vi "Check mtcdt check cell radio.vi"(6 "VISA resource name":refnum<visa-resource-name>="COM5", 7 "Passed so far":bool, 8 "error in (no error)":errorcluster, 9 "RadioType":T2) -> (0 "error out":errorcluster, 2 "imei":string, 3 "Radio info":T1, 4 "VISA Refnum out":refnum<visa-resource-name>, 5 "Passed?":bool)   [LabVIEW 2024]
uses:
  MTCDT_radio_type.ctl
panel:
  in  "Temp config":string
  in  "FW Build":string
  in  "TelitModuleVer":string
  in  "RadioVersion":string
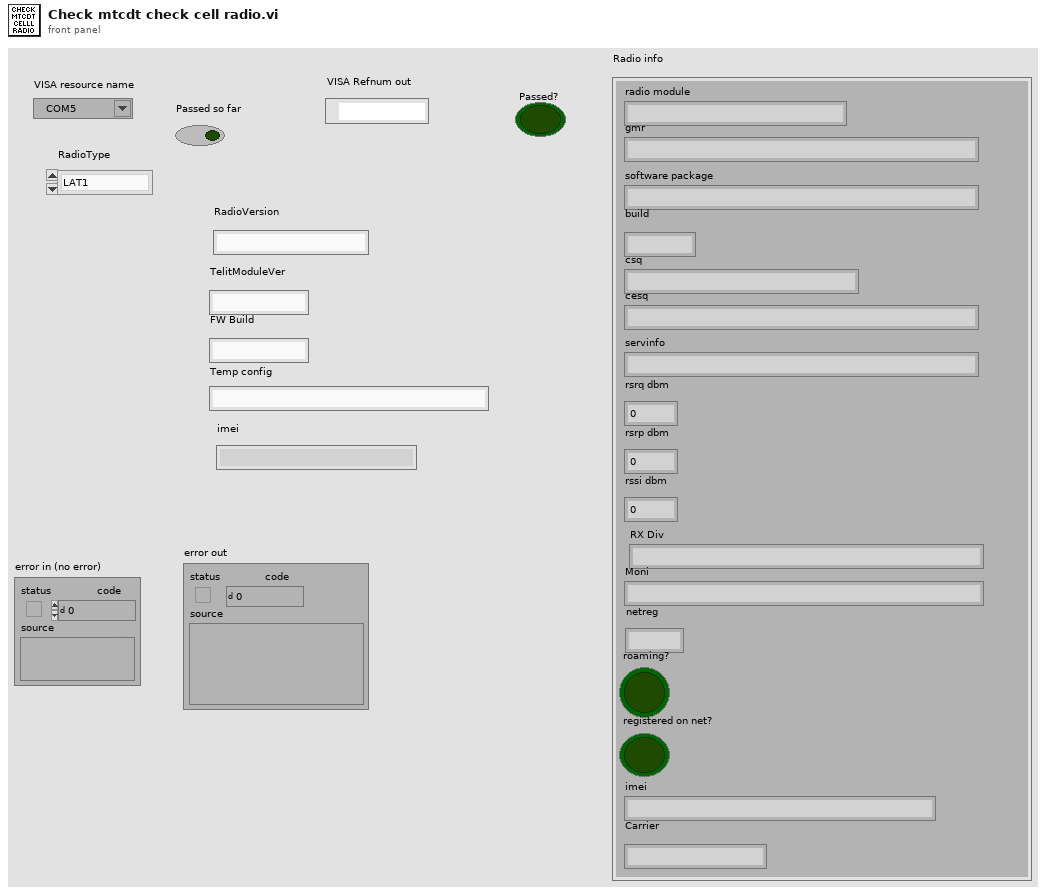
[diagram p1: front panel]
types:
  T1 = cluster{"radio module":string, "gmr":string, "software package":string, "csq":string, "cesq":string, "servinfo":string, "rsrq dbm":dbl, "rsrp dbm":dbl, "rssi dbm":dbl, "build":string, "RX Div":string, "Moni":string, "netreg":string, "roaming?":bool, "registered on net?":bool, "imei":string, "Carrier":string}
  T2 = typedef "MTCDT_radio_type.ctl" = enum16{"LAT1", "H5", "LAT3", "LEU1", "L4E1", "L4N1", "LVW2", "LSB3", "LDC3", "LAP3", "L4G1", "L6G1"}
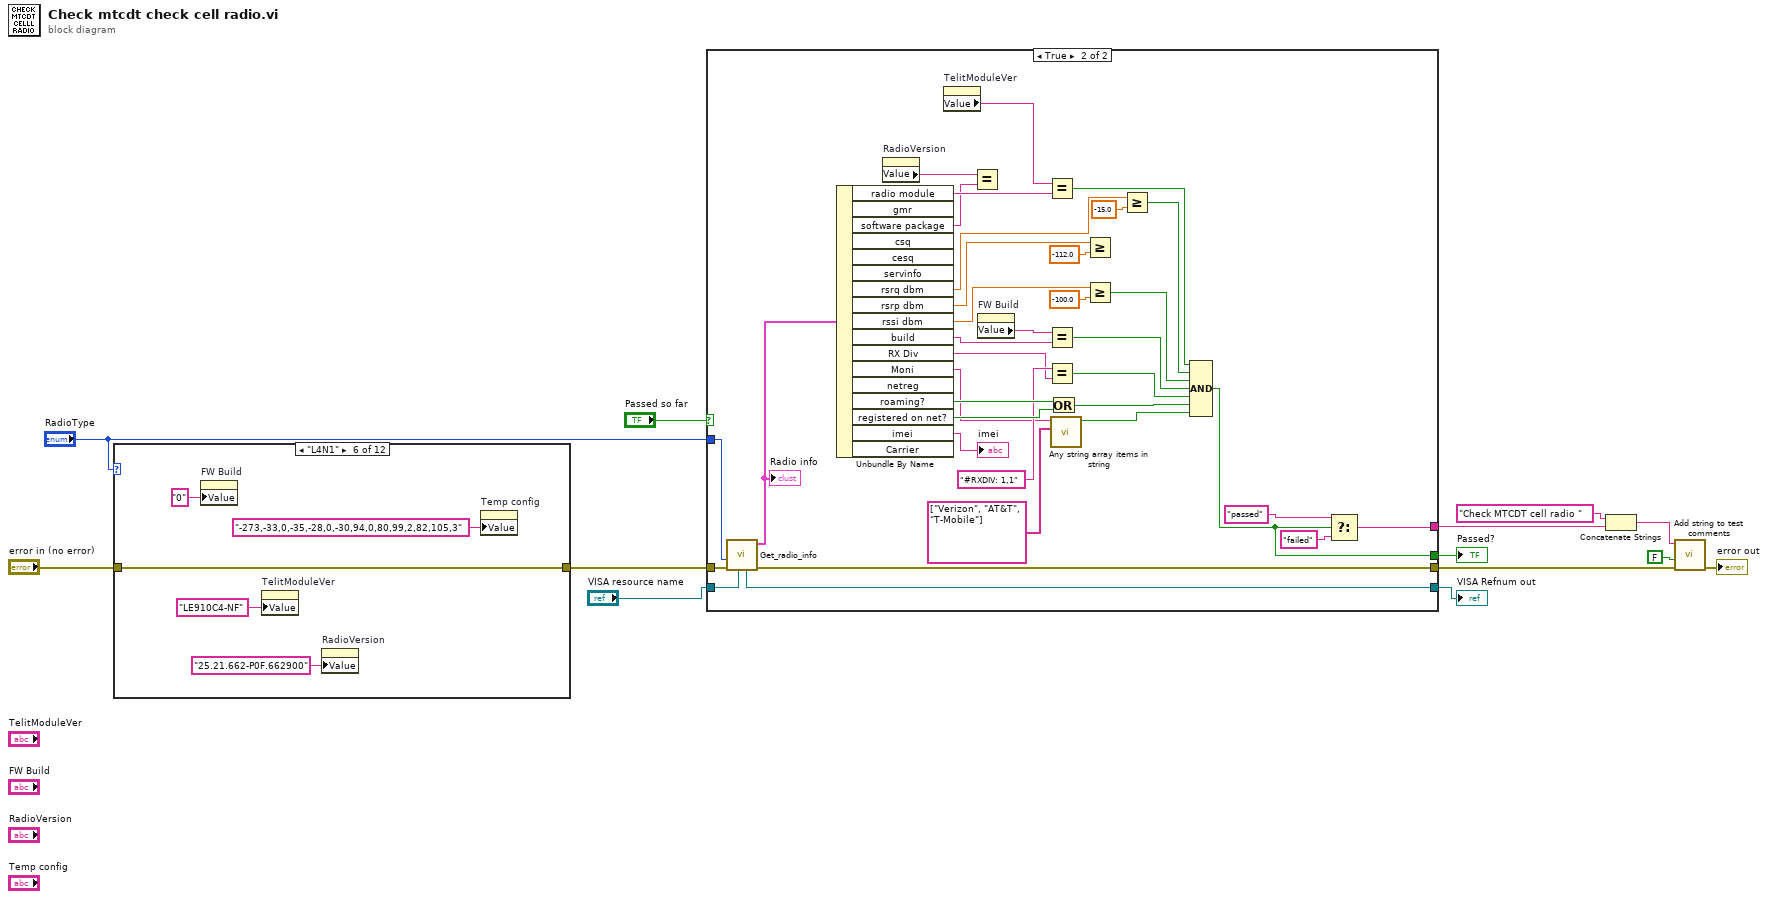
[diagram p0: block diagram]
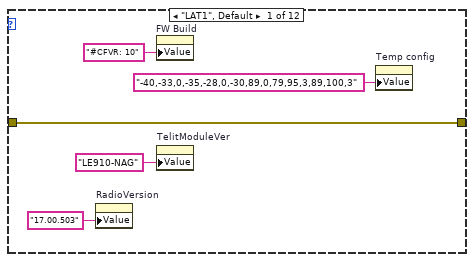
[diagram p2: hidden frame]
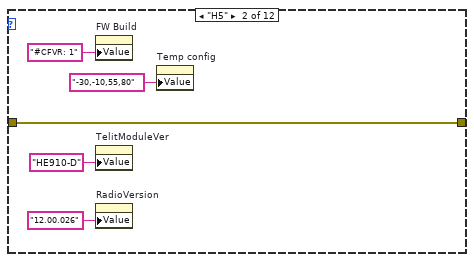
[diagram p3: hidden frame]
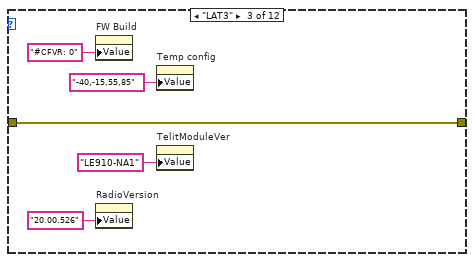
[diagram p4: hidden frame]
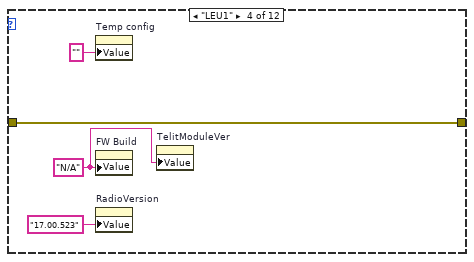
[diagram p5: hidden frame]
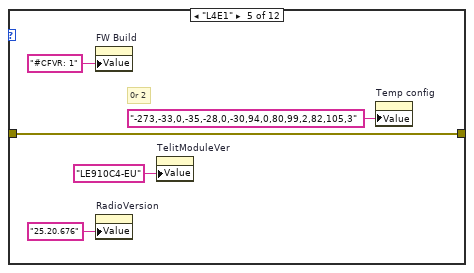
[diagram p6: hidden frame]
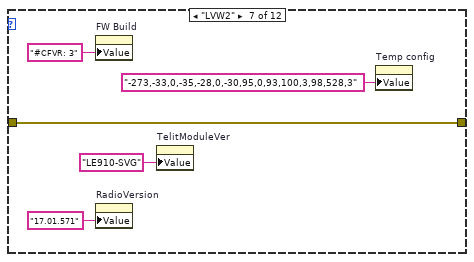
[diagram p7: hidden frame]
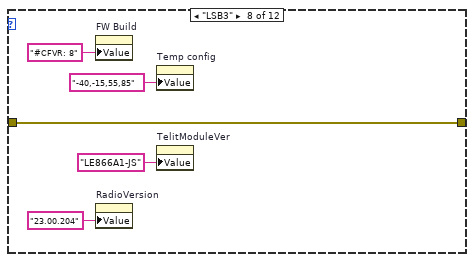
[diagram p8: hidden frame]
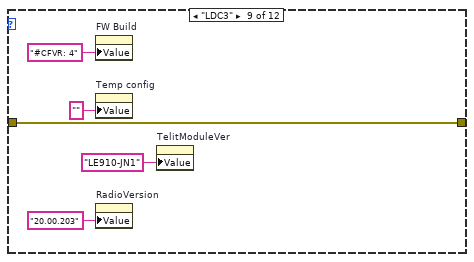
[diagram p9: hidden frame]
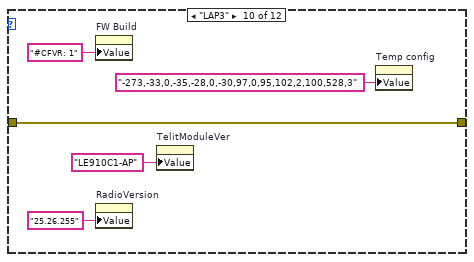
[diagram p10: hidden frame]
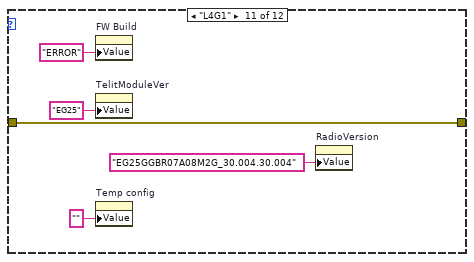
[diagram p11: hidden frame]
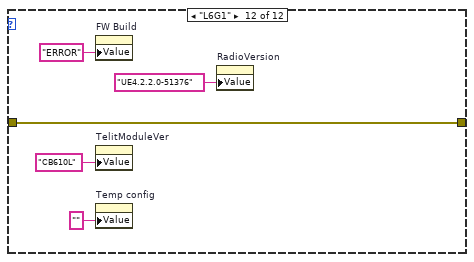
[diagram p12: hidden frame]
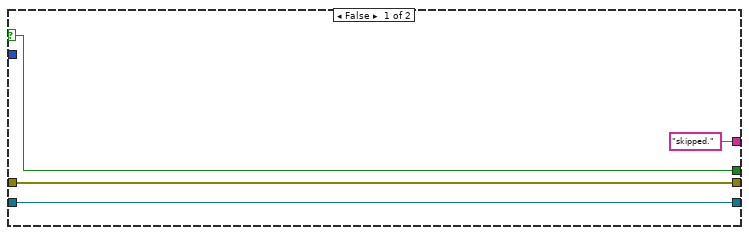
[diagram p13: hidden frame]
diagram:
  n1 = case shown="\"L4N1\"" "RadioType" {
    tunnel: [w14 w19 w24 w29 w33 w38 w43 w48 w53 w58 w63 w68] -> w4
    tunnel: "error in (no error)" -> [w14 w19 w24 w29 w33 w38 w43 w48 w53 w58 w63 w68]
    frame "LAT1", Default {
      n2 = property on="RadioVersion" class="Str"("Value"="17.00.503" ("RadioVersion")) -> ()  [unwired: 2 in, 2 out]
      n3 = property on="FW Build" class="Str"("Value"="#CFVR: 10" ("FW Build")) -> ()  [unwired: 2 in, 2 out]
      n4 = property on="TelitModuleVer" class="Str"("Value"="LE910-NAG" ("TelitModuleVer")) -> ()  [unwired: 2 in, 2 out]
      n5 = property on="Temp config" class="Str"("Value"="-40,-33,0,-35,-28,0,-30,89,0,79,95,3,89,100,3" ("Temp config")) -> ()  [unwired: 2 in, 2 out]
    }
    frame "H5" {
      n6 = property on="FW Build" class="Str"("Value"="#CFVR: 1" ("FW Build")) -> ()  [unwired: 2 in, 2 out]
      n7 = property on="TelitModuleVer" class="Str"("Value"="HE910-D" ("TelitModuleVer")) -> ()  [unwired: 2 in, 2 out]
      n8 = property on="RadioVersion" class="Str"("Value"="12.00.026" ("RadioVersion")) -> ()  [unwired: 2 in, 2 out]
      n9 = property on="Temp config" class="Str"("Value"="-30,-10,55,80" ("Temp config")) -> ()  [unwired: 2 in, 2 out]
    }
    frame "LAT3" {
      n10 = property on="FW Build" class="Str"("Value"="#CFVR: 0" ("FW Build")) -> ()  [unwired: 2 in, 2 out]
      n11 = property on="RadioVersion" class="Str"("Value"="20.00.526" ("RadioVersion")) -> ()  [unwired: 2 in, 2 out]
      n12 = property on="Temp config" class="Str"("Value"="-40,-15,55,85" ("Temp config")) -> ()  [unwired: 2 in, 2 out]
      n13 = property on="TelitModuleVer" class="Str"("Value"="LE910-NA1" ("TelitModuleVer")) -> ()  [unwired: 2 in, 2 out]
    }
    frame "LEU1" {
      w31 = "N/A" ("TelitModuleVer")
      n14 = property on="Temp config" class="Str"("Value"="" ("Temp config")) -> ()  [unwired: 2 in, 2 out]
      n15 = property on="FW Build" class="Str"("Value"=w31) -> ()  [unwired: 2 in, 2 out]
      n16 = property on="RadioVersion" class="Str"("Value"="17.00.523" ("RadioVersion")) -> ()  [unwired: 2 in, 2 out]
      n17 = property on="TelitModuleVer" class="Str"("Value"=w31) -> ()  [unwired: 2 in, 2 out]
    }
    frame "L4E1" {
      # "0r 2"
      n18 = property on="FW Build" class="Str"("Value"="#CFVR: 1" ("FW Build")) -> ()  [unwired: 2 in, 2 out]
      n19 = property on="RadioVersion" class="Str"("Value"="25.20.676" ("RadioVersion")) -> ()  [unwired: 2 in, 2 out]
      n20 = property on="TelitModuleVer" class="Str"("Value"="LE910C4-EU" ("TelitModuleVer")) -> ()  [unwired: 2 in, 2 out]
      n21 = property on="Temp config" class="Str"("Value"="-273,-33,0,-35,-28,0,-30,94,0,80,99,2,82,105,3" ("Temp config")) -> ()  [unwired: 2 in, 2 out]
    }
    frame "L4N1" {
      n22 = property on="FW Build" class="Str"("Value"="0" ("FW Build")) -> ()  [unwired: 2 in, 2 out]
      n23 = property on="TelitModuleVer" class="Str"("Value"="LE910C4-NF" ("TelitModuleVer")) -> ()  [unwired: 2 in, 2 out]
      n24 = property on="RadioVersion" class="Str"("Value"="25.21.662-P0F.662900" ("RadioVersion")) -> ()  [unwired: 2 in, 2 out]
      n25 = property on="Temp config" class="Str"("Value"="-273,-33,0,-35,-28,0,-30,94,0,80,99,2,82,105,3" ("Temp config")) -> ()  [unwired: 2 in, 2 out]
    }
    frame "LVW2" {
      n26 = property on="FW Build" class="Str"("Value"="#CFVR: 3" ("FW Build")) -> ()  [unwired: 2 in, 2 out]
      n27 = property on="RadioVersion" class="Str"("Value"="17.01.571" ("RadioVersion")) -> ()  [unwired: 2 in, 2 out]
      n28 = property on="TelitModuleVer" class="Str"("Value"="LE910-SVG" ("TelitModuleVer")) -> ()  [unwired: 2 in, 2 out]
      n29 = property on="Temp config" class="Str"("Value"="-273,-33,0,-35,-28,0,-30,95,0,93,100,3,98,528,3" ("Temp config")) -> ()  [unwired: 2 in, 2 out]
    }
    frame "LSB3" {
      n30 = property on="FW Build" class="Str"("Value"="#CFVR: 8" ("FW Build")) -> ()  [unwired: 2 in, 2 out]
      n31 = property on="RadioVersion" class="Str"("Value"="23.00.204" ("RadioVersion")) -> ()  [unwired: 2 in, 2 out]
      n32 = property on="Temp config" class="Str"("Value"="-40,-15,55,85" ("Temp config")) -> ()  [unwired: 2 in, 2 out]
      n33 = property on="TelitModuleVer" class="Str"("Value"="LE866A1-JS" ("TelitModuleVer")) -> ()  [unwired: 2 in, 2 out]
    }
    frame "LDC3" {
      n34 = property on="FW Build" class="Str"("Value"="#CFVR: 4" ("FW Build")) -> ()  [unwired: 2 in, 2 out]
      n35 = property on="Temp config" class="Str"("Value"="" ("Temp config")) -> ()  [unwired: 2 in, 2 out]
      n36 = property on="RadioVersion" class="Str"("Value"="20.00.203" ("RadioVersion")) -> ()  [unwired: 2 in, 2 out]
      n37 = property on="TelitModuleVer" class="Str"("Value"="LE910-JN1" ("TelitModuleVer")) -> ()  [unwired: 2 in, 2 out]
    }
    frame "LAP3" {
      n38 = property on="FW Build" class="Str"("Value"="#CFVR: 1" ("FW Build")) -> ()  [unwired: 2 in, 2 out]
      n39 = property on="RadioVersion" class="Str"("Value"="25.26.255" ("RadioVersion")) -> ()  [unwired: 2 in, 2 out]
      n40 = property on="TelitModuleVer" class="Str"("Value"="LE910C1-AP" ("TelitModuleVer")) -> ()  [unwired: 2 in, 2 out]
      n41 = property on="Temp config" class="Str"("Value"="-273,-33,0,-35,-28,0,-30,97,0,95,102,2,100,528,3" ("Temp config")) -> ()  [unwired: 2 in, 2 out]
    }
    frame "L4G1" {
      n42 = property on="FW Build" class="Str"("Value"="ERROR" ("FW Build")) -> ()  [unwired: 2 in, 2 out]
      n43 = property on="TelitModuleVer" class="Str"("Value"="EG25" ("TelitModuleVer")) -> ()  [unwired: 2 in, 2 out]
      n44 = property on="Temp config" class="Str"("Value"="" ("Temp config")) -> ()  [unwired: 2 in, 2 out]
      n45 = property on="RadioVersion" class="Str"("Value"="EG25GGBR07A08M2G_30.004.30.004" ("RadioVersion")) -> ()  [unwired: 2 in, 2 out]
    }
    frame "L6G1" {
      n46 = property on="FW Build" class="Str"("Value"="ERROR" ("FW Build")) -> ()  [unwired: 2 in, 2 out]
      n47 = property on="TelitModuleVer" class="Str"("Value"="CB610L" ("TelitModuleVer")) -> ()  [unwired: 2 in, 2 out]
      n48 = property on="Temp config" class="Str"("Value"="" ("Temp config")) -> ()  [unwired: 2 in, 2 out]
      n49 = property on="RadioVersion" class="Str"("Value"="UE4.2.2.0-51376" ("RadioVersion")) -> ()  [unwired: 2 in, 2 out]
    }
  }
  n50 = case shown="True" "Passed so far" {
    selector: "Passed so far" -> [w76 _]
    tunnel: w4 -> [w75 w112]
    tunnel: [w75 w108] -> w5
    tunnel: "VISA resource name" -> [w74 w110]
    tunnel: [w76 w78] -> w8
    tunnel: [w74 w109] -> w6
    tunnel: "RadioType" -> [_ w111]
    tunnel: ["skipped." w77] -> w1
    frame False {
    }
    frame True {
      n51 = call "Get_radio_info.vi"("VISA resource name"=w110, "error in (no error)"=w112, "RadioType"=w111) -> ("error out"=w108:errorcluster, "Radio info"=w107:T1, "VISA resource name out"=w109:refnum<visa-resource-name>)  [unwired: 5 in, 1 out]
      "Radio info" <- w107
      n52 = Unbundle By Name(w107) -> ("radio module"=w105:string, "software package"=w103:string, "rsrq dbm"=w92:dbl, "rsrp dbm"=w94:dbl, "rssi dbm"=w96:dbl, "build"=w101:string, "RX Div"=w97:string, "Moni"=w89:string, "roaming?"=w100:bool, "registered on net?"=w99:bool, "imei"=→"imei":string)  [unwired: 6 out]
      n53 = property on="RadioVersion" class="Str"() -> ("Value"=w104:string)  [unwired: 2 in, 2 out]
      n54 = property on="TelitModuleVer" class="Str"() -> ("Value"=w106:string)  [unwired: 2 in, 2 out]
      n55 = Equal?(x=w104, y=w103) -> ()  [unwired: 1 out]
      n56 = property on="FW Build" class="Str"() -> ("Value"=w102:string)  [unwired: 2 in, 2 out]
      n57 = Equal?(x=w106, y=w105) -> (x = y?=w87:bool)
      n58 = Equal?(x=w102, y=w101) -> (x = y?=w84:bool)
      n59 = Equal?(x="#RXDIV: 1,1", y=w97) -> (x = y?=w83:bool)
      n60 = Or(x=w100, y=w99) -> (x .or. y?=w82:bool)
      n61 = call "Any string array items in string.vi"("Strings to look for"=string[] ["Verizon", "AT&T", "T-Mobile"], "String buffer"=w89) -> ("In string?"=w81:bool)  [unwired: 8 in, 1 out]
      n62 = Greater Or Equal?(x=w94, y=-112.0) -> ()  [unwired: 1 out]
      n63 = Greater Or Equal?(x=w96, y=-100.0) -> (x >= y?=w85:bool)
      n64 = Greater Or Equal?(x=w92, y=-15.0) -> (x >= y?=w86:bool)
      n65 = Compound Arithmetic op=AND(w87, w86, w85, w84, w83, w82, w81) -> (w78:bool)
      n66 = Select(t="passed", s=w78, f="failed") -> (s? t:f=w77:string)
    }
  }
  "Passed?" <- w8
  "VISA Refnum out" <- w6
  n67 = Concatenate Strings("Check MTCDT cell radio " ("string"), w1) -> (w11:string)
  n68 = call "Add string to test comments.vi"("error in (no error)"=w5, "New Section (y)?"=FALSE, "Comments"=w11) -> ("error out"=→"error out":errorcluster)  [unwired: 7 in, 1 out]
